vi "proc.util.compare-function.vi"(8 "error in (no error)":errorcluster, 10 "input cluster":cluster{"Comparison":string, "Setpoint":dbl}, 11 "Input":dbl) -> (0 "error out":errorcluster, 2 "String":string, 3 "Result Condition":bool)   [LabVIEW 2024]
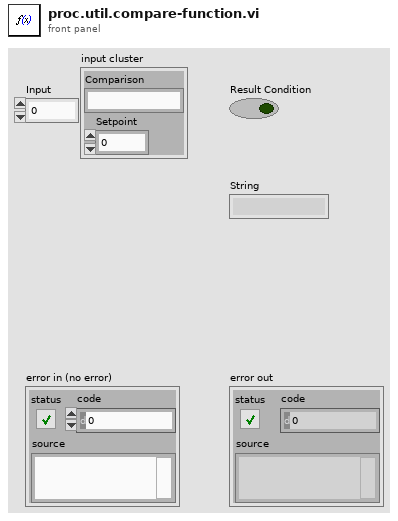
[diagram p1: front panel]
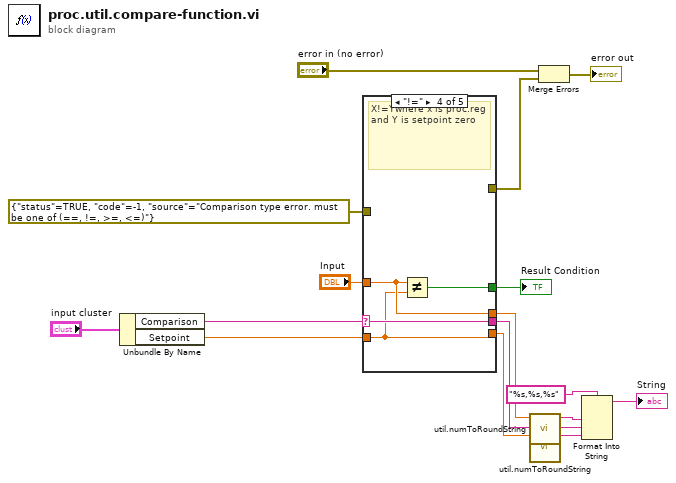
[diagram p0: block diagram]
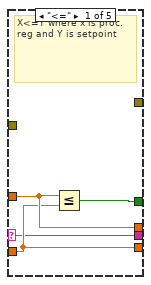
[diagram p2: hidden frame]
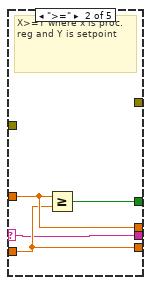
[diagram p3: hidden frame]
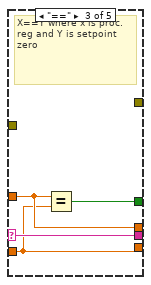
[diagram p4: hidden frame]
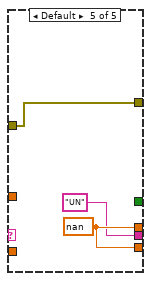
[diagram p5: hidden frame]
diagram:
  n1 = Unbundle By Name("input cluster") -> ("Comparison"=w2:string, "Setpoint"=w1:dbl)
  n2 = case shown="\"!=\"" w2 {
    selector: w2 -> [w17 w21 w27 w30 _]
    tunnel: [w20 w24 w28 w32 _] -> w4
    tunnel: "Input" -> [w19 w23 w26 w31 _]
    tunnel: w1 -> [w18 w22 w25 w29 _]
    tunnel: [w19 w23 w26 w31 w34] -> w11
    tunnel: [w17 w21 w27 w30 "UN"] -> w6
    tunnel: [w18 w22 w25 w29 w34] -> w13
    tunnel: errorcluster {"status"=TRUE, "code"=-1, "source"="Comparison type error. must be one of (==, !=, >=, <=)"} ("error out") -> [_ _ _ _ w35]
    tunnel: [_ _ _ _ w35] -> w9
    frame "<=" {
      # "X<=Y where x is proc.reg and Y is setpoint"
      n3 = Less Or Equal?(x=w19, y=w18) -> (x <= y?=w20:bool)
    }
    frame ">=" {
      # "X>=Y where x is proc.reg and Y is setpoint"
      n4 = Greater Or Equal?(x=w23, y=w22) -> (x >= y?=w24:bool)
    }
    frame "==" {
      # "X==Y where x is proc.reg and Y is setpoint zero"
      n5 = Equal?(x=w26, y=w25) -> (x = y?=w28:bool)
    }
    frame "!=" {
      # "X!=Ywhere x is proc.reg and Y is setpoint zero"
      n6 = Not Equal?(x=w31, y=w29) -> (x != y?=w32:bool)
    }
    frame Default {
      w34 = nan ("reg in")
    }
  }
  "Result Condition" <- w4
  n7 = call "util.numToRoundString.vi"("reg in"=w11) -> ("String"=w12:string)  [unwired: 10 in]
  n8 = call "util.numToRoundString.vi"("reg in"=w13) -> ("String"=w14:string)  [unwired: 10 in]
  n9 = Merge Errors("error in (no error)", w9) -> (→"error out":errorcluster)
  n10 = Format Into String(format string="%s,%s,%s", w12, w6, w14) -> (resulting string=→"String":string)  [unwired: 2 in, 1 out]
